vi "UE9 Hardware Counter Example.vi"() -> ()   [LabVIEW 2021]
panel:
  out "Counter Reads":u32[](array[numeric])
  in  "Reset Counters":bool
  in  "Iteration Inverval (ms)":u32=100
  out "Iteration":i32
  in  "error in":errorcluster
  in  "ConnectionType":u16(ring) items=["LJ_ctUSB", "LJ_ctETHERNET"]
  in  "Address":string="1"
  in  "FirstFound":bool=TRUE
  in  "stop":bool
  out "error out":errorcluster
  out "Error Message":string
  # "Enables both hardware counters, then reads them at the specified interval.\nSince there are no timers enabled, Counter0 will be on FIO0 nd Counter1 will be on FIO1."
  # "Counter0"
  # "Counter1"
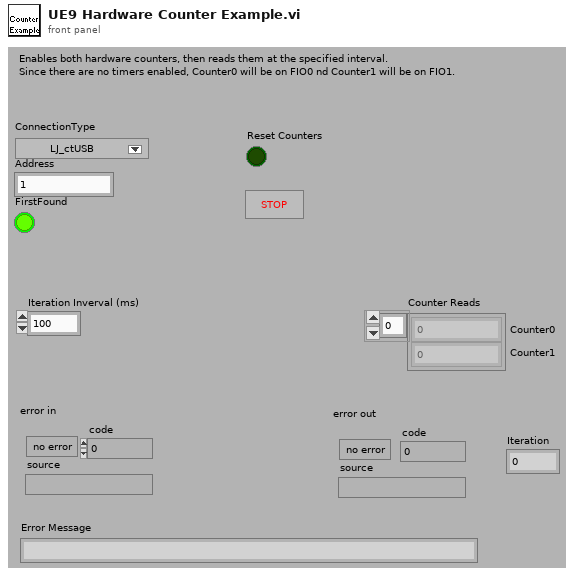
[diagram p1: front panel]
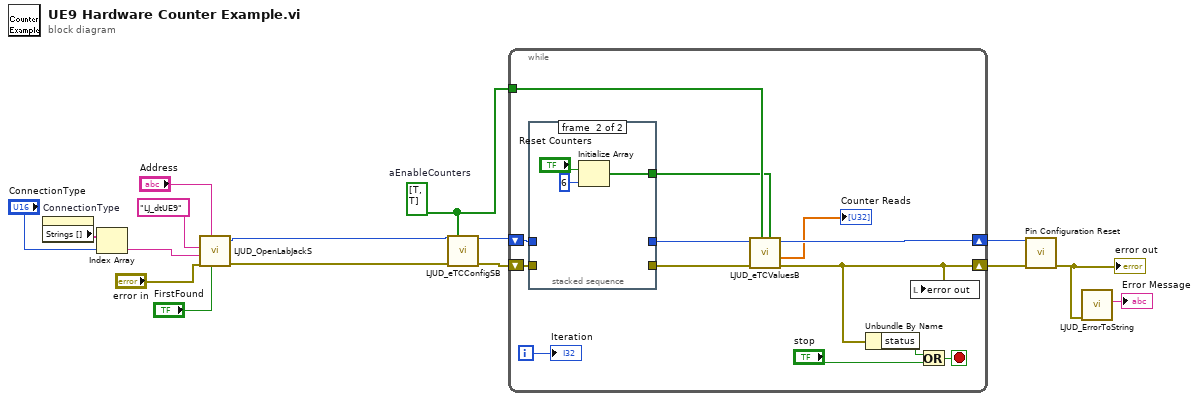
[diagram p0: block diagram]
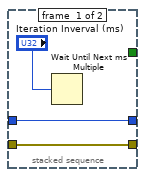
[diagram p2: hidden frame]
diagram:
  w1 = bool[] [TRUE, TRUE]  # aEnableCounters
  n1 = property on="ConnectionType" class="Ring (strict)"() -> ("Strings []"=w11:string[])  [unwired: 2 in, 2 out]
  n2 = Index Array(array=w11, index="ConnectionType") -> (element=w9:string)
  n3 = call "LJUD_OpenLabJackS.vi"("FirstFound"="FirstFound", "Address"="Address", "error in"="error in", "ConnectionType"=w9, "DeviceType"="LJ_dtUE9") -> ("error out"=w3:errorcluster, "Handle"=w2:i32)  [unwired: 4 in, 1 out]
  n4 = call "LJUD_eTCConfigSB.vi"("Handle In"=w2, "aEnableCounters"=w1, "error in"=w3) -> ("Handle Out"=w7:i32, "error out"=w8:errorcluster)  [unwired: 11 in]
  n5 = while {
    tunnel: w1 -> [w20]
    shift-left: w8 -> [w28]
    shift-right: [w17] -> w5
    shift-left: w7 -> [w29]
    shift-right: [w21] -> w6
    i -> [w22]
    stop <- w25 stop-if-true
    n6 = stacked-sequence {
      tunnel: [w32 _] -> w27
      tunnel: [w31 _] -> w26
      tunnel: w29 -> [w32 _]
      tunnel: w28 -> [w31 _]
      tunnel: [_ w33] -> w19
      frame #0 {
        n7 = Wait Until Next ms Multiple(millisecond multiple="Iteration Inverval (ms)") -> ()  [unwired: 1 out]
      }
      frame #1 {
        n8 = Initialize Array("Reset Counters", 6 ("Dimension Size")) -> (w33:bool[])
      }
    }
    n9 = call "LJUD_eTCValuesB.vi"("aResetCounters"=w19, "aReadCounters"=w20, "error in"=w26, "Handle In"=w27) -> ("error out"=w17:errorcluster, "aCounterValues"=→"Counter Reads":dbl[], "Handle Out"=w21:i32)  [unwired: 4 in, 1 out]
    n10 = Unbundle By Name(w17) -> ("status"=w24:bool)
    n11 = local write "error out"(w17) -> ()
    n12 = Or(x=w24, y="stop") -> (x .or. y?=w25:bool)
    "Iteration" <- w22
  }
  n13 = call "Pin Configuration Reset.vi"("error in"=w5, "Handle In"=w6) -> ("error out"=w4:errorcluster)  [unwired: 8 in, 1 out]
  "error out" <- w4
  n14 = call "LJUD_ErrorToString.vi"("error in"=w4) -> ("String"=→"Error Message":string)  [unwired: 10 in]
